vi "dfd_CIC_CombDummy.vi"(10 "input valid":bool=TRUE, 11 "data in":bool[](array[boolean])) -> (0 "ready for input":bool, 2 "output valid":bool, 3 "data out":bool[](array[boolean]))   [LabVIEW 2017]
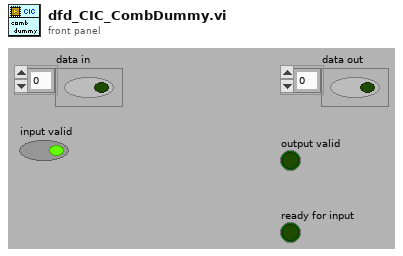
[diagram p1: front panel]
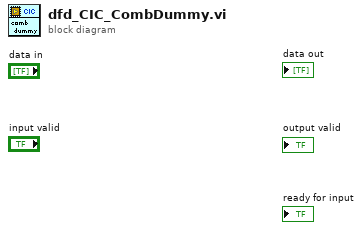
[diagram p0: block diagram]
diagram:
